vi "teste_comunicação.vi"() -> ()   [LabVIEW 2019]
panel:
  out "error out 2":errorcluster
  out "error out":errorcluster
  in  "stop":bool
  out "Intel out":u8
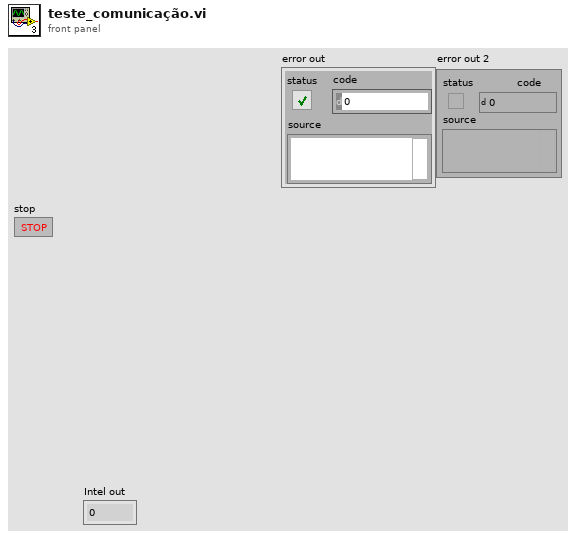
[diagram p1: front panel]
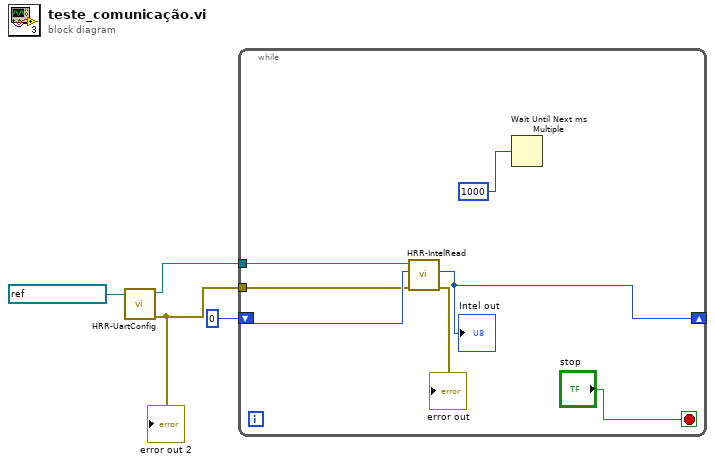
[diagram p0: block diagram]
diagram:
  n1 = call "HRR-UartConfig.vi"("VISA resource name in"=refnum<visa-resource-name> "ASRL2::INSTR") -> ("error out"=w1:errorcluster, "VISA resource name out"=w3:refnum<visa-resource-name>)  [unwired: 9 in]
  "error out 2" <- w1
  n2 = while {
    tunnel: w3 -> [w11]
    shift-right: [w9] -> _
    shift-left: u8 0 -> [w10]
    tunnel: w1 -> [w6]
    stop <- "stop" stop-if-true
    n3 = call "HRR-IntelRead.vi"("error in (no error)"=w6, "Intel in"=w10, "VISA resource name in"=w11) -> ("error out"=→"error out":errorcluster, "Intel out"=w9:u8)  [unwired: 6 in, 1 out]
    "Intel out" <- w9
    n4 = Wait Until Next ms Multiple(millisecond multiple=u32 1000) -> ()  [unwired: 1 out]
  }
